vi "Client.vi"() -> ()   [LabVIEW 2021]
panel:
  in  "Button":bool
  out "error out":errorcluster
  out "Image":T1(plugin-control)
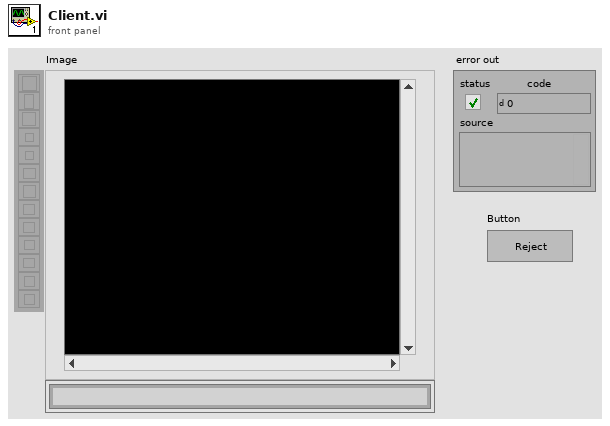
[diagram p1: front panel]
types:
  T1 = typedef "IMAQ Image.ctl" = refnum<image>
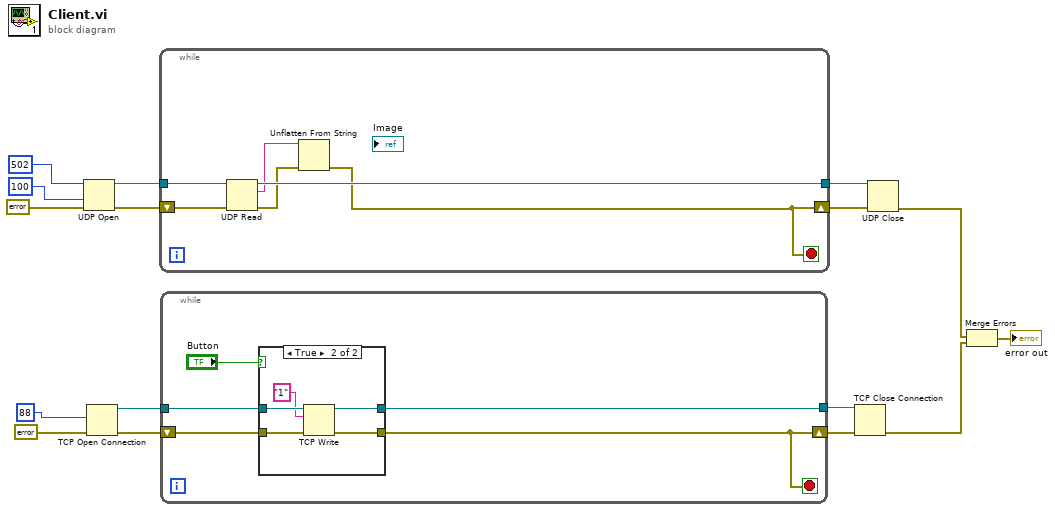
[diagram p0: block diagram]
diagram:
  n1 = UDP Open(8:errorcluster {"status"=FALSE, "code"=0, "source"=""} ("error in (no error)"), 9:100 ("timeout ms (25000)"), 11:u16 502 ("port")) -> (port=w13:refnum<k16>, 0:w16:errorcluster)  [unwired: 2 in, 1 out]
  n2 = TCP Open Connection(remote port or service name=u16 88, error in (no error)=errorcluster {"status"=FALSE, "code"=0, "source"=""}) -> (connection ID=w7:refnum<k5>, error out=w10:errorcluster)  [unwired: 3 in]
  n3 = while {
    shift-right: [w18] -> w12
    shift-left: w16 -> [w22]
    tunnel: w13 -> [w21]
    tunnel: [w20] -> w11
    stop <- w18 stop-if-true
    n4 = UDP Read(connection ID=w21, 8:w22) -> (data out=w17:string, error out=w19:errorcluster, 3:w20:refnum<k16>)  [unwired: 2 in, 2 out]
    n5 = Unflatten From String(binary string=w17, error in (no error)=w19) -> (error out=w18:errorcluster)  [unwired: 3 in, 2 out]
  }
  n6 = while {
    shift-right: [w25] -> w6
    shift-left: w10 -> [w24]
    tunnel: w7 -> [w23]
    tunnel: [w26] -> w5
    stop <- w25 stop-if-true
    n7 = case shown="True" "Button" {
      tunnel: [w29 w34] -> w26
      tunnel: [w28 w33] -> w25
      tunnel: w24 -> [w28 w32]
      tunnel: w23 -> [w29 w31]
      frame False {
      }
      frame True {
        n8 = TCP Write(connection ID=w31, data in="1", error in (no error)=w32) -> (connection ID out=w34:refnum<k5>, error out=w33:errorcluster)  [unwired: 1 in, 1 out]
      }
    }
  }
  n9 = TCP Close Connection(connection ID=w5, error in (no error)=w6) -> (error out=w2:errorcluster)  [unwired: 1 in, 1 out]
  n10 = UDP Close(connection ID=w11, 8:w12) -> (error out=w3:errorcluster)  [unwired: 1 out]
  n11 = Merge Errors(w3, w2) -> (→"error out":errorcluster)
